vi "build_1d_scan_voltage_arrays.vi"(6 "y end":i32, 7 "y start":i32, 9 "scan points":i32, 10 "x start":i32, 11 "x end":i32) -> (2 "y voltage array":dbl[](array[numeric]), 3 "x voltage array":dbl[](array[numeric]))   [LabVIEW 2022 SP3]
uses:
  <vilib>/Analysis/1siggen.llb/Ramp Pattern by Samples.vi
  <vilib>/Analysis/NI_AALBase.lvlib
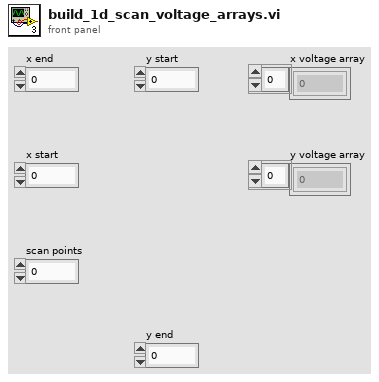
[diagram p1: front panel]
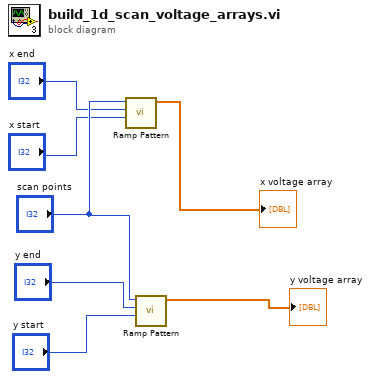
[diagram p0: block diagram]
diagram:
  n1 = call-poly <vilib>:"Ramp Pattern.vi"("start"="x start", "end"="x end", "samples"="scan points") -> ("Ramp Pattern"=→"x voltage array":dbl[])  [unwired: 7 in, 1 out]
  n2 = call-poly <vilib>:"Ramp Pattern.vi"("start"="y start", "end"="y end", "samples"="scan points") -> ("Ramp Pattern"=→"y voltage array":dbl[])  [unwired: 7 in, 1 out]
